vi "CycleX.vi"(0 "Devices queue":refnum<queue>, 1 "Program only changes":bool, 5 "Program during MOT loading":bool, 7 "Igor Inform String":string[](array[string]), 9 "Additional wait time (s)":dbl, 11 "error in":errorcluster) -> (8 "error out":errorcluster)   [LabVIEW 2013]
uses:
  Device/Device.lvclass
  Master Device/Master Device.lvclass
  Globals/Total Time.vi
panel:
  # "Status and timing"
  # "Igor options"
  # "Hardware control"
  # "This option starts the pulse blaster and then programs the external devices.  If the MOT loading time is not long enough for this process to complete there will be problems."
  # "When set, this option only\nasks a device to program\nitself if it's hardware image\nhas actually changed."
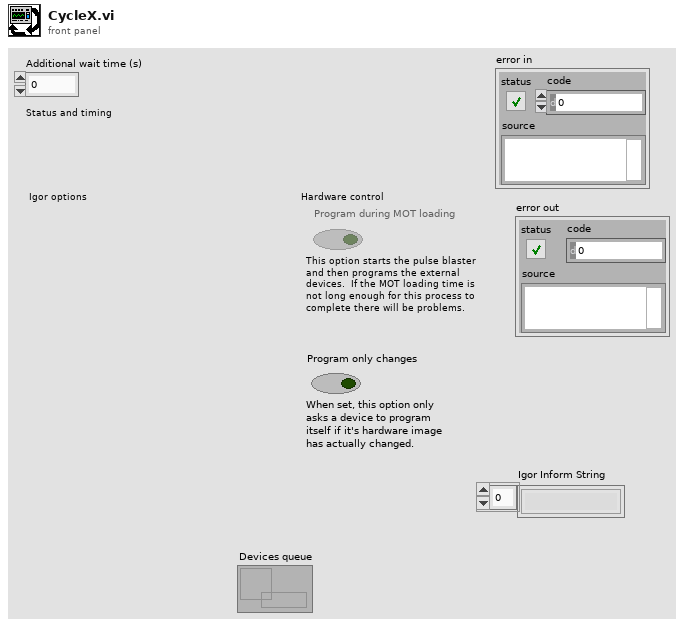
[diagram p1: front panel]
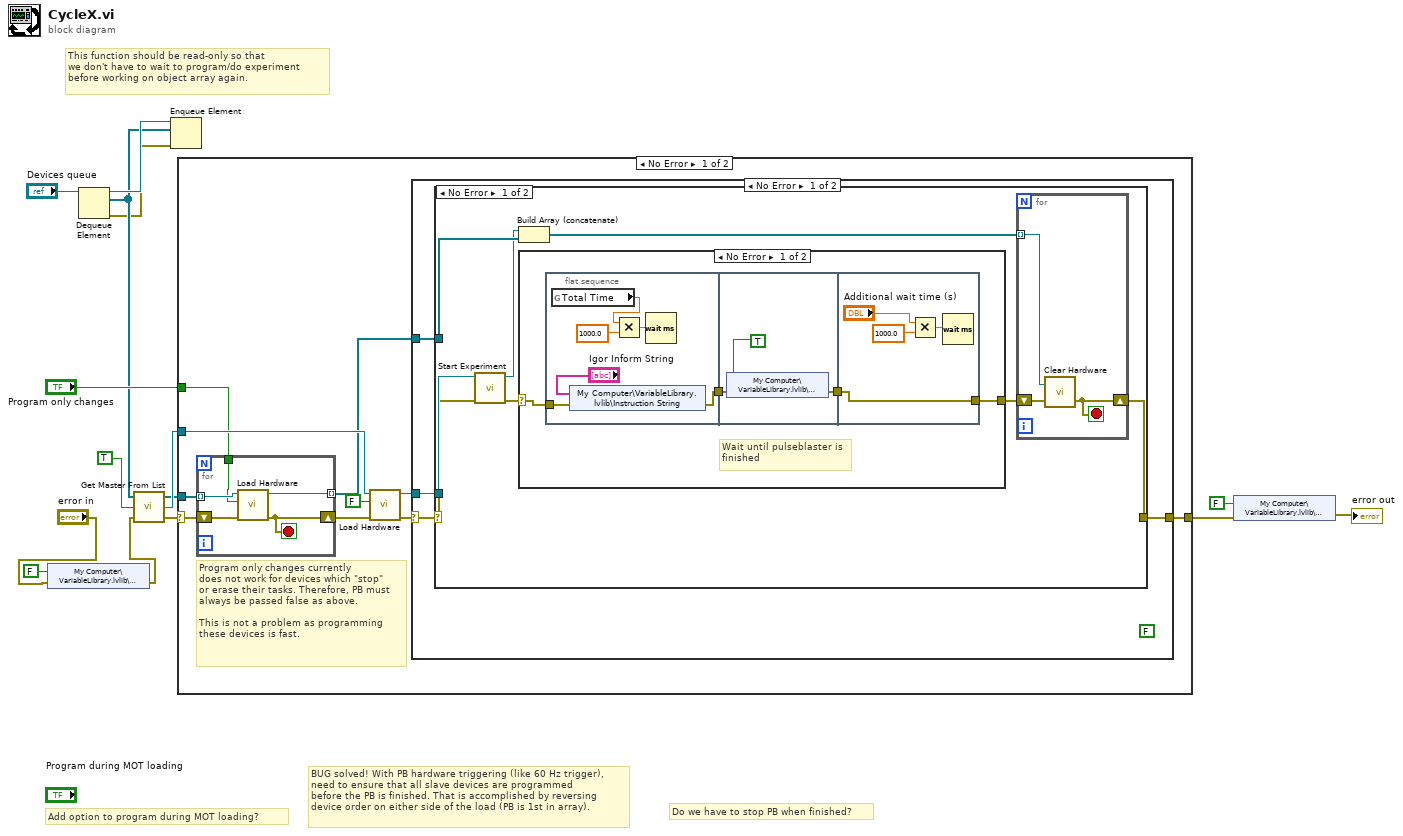
[diagram p0: block diagram]
diagram:
  # "This function should be read-only so that \nwe don't have to wait to program/do experiment \nbefore working on object array again."
  # "BUG solved! With PB hardware triggering (like 60 Hz trigger),\nneed to ensure that all slave devices are programmed\nbefore the PB is finished. That is accomplished by reversing\ndevice order on either side of the load (PB is 1st in array)."
  # "Do we have to stop PB when finished?"
  # "Add option to program during MOT loading?"
  n1 = shared-variable "My Computer\\VariableLibrary.lvlib\\CycleDone"(FALSE ("CycleDone"), error in="error in") -> (error out=w7:errorcluster)
  n2 = Dequeue Element(queue="Devices queue") -> (queue out=w10:refnum<queue>, element=w9:refnum<class "Device.lvclass">[], error out=w8:errorcluster)  [unwired: 2 in, 1 out]
  n3 = call "Get Master From List.vi"("error in"=w7, "Del From List?"=TRUE, "Device List in"=w9) -> ("error out"=w12:errorcluster, "Master Device"=w14:refnum<class "Master Device.lvclass">, "Device List out"=w13:refnum<class "Device.lvclass">[])
  n4 = Enqueue Element(queue=w10, element=w9, error in (no error)=w8) -> ()  [unwired: 1 in, 3 out]
  n5 = case shown="No Error" w12 {
    selector: w12 -> [w20 w66]
    tunnel: w14 -> [w24 _]
    tunnel: w13 -> [w23 _]
    tunnel: [w19 w66] -> w3
    tunnel: "Program only changes" -> [w17 _]
    frame No Error {
      # "Program only changes currently\ndoes not work for devices which \"stop\"\nor erase their tasks. Therefore, PB must\nalways be passed false as above.\n\nThis is not a problem as programming\nthese devices is fast."
      n6 = for {
        tunnel: w23 -> [w65] mode=indexing
        shift-right: [w63] -> w25
        shift-left: w20 -> [w64]
        tunnel: [w62] -> w22 mode=indexing
        tunnel: w17 -> [w61]
        stop <- w63 stop-if-true
        n7 = call-dynamic "Load Hardware.vi"("error in (no error)"=w64, "Program only changes"=w61, "Device in"=w65) -> ("error out"=w63:errorcluster, "Device out"=w62:refnum<class "Device.lvclass">)  [unwired: 7 in]
      }
      n8 = call-dynamic "Load Hardware.vi"("error in (no error)"=w25, "Program only changes"=FALSE, "Master Device in"=w24) -> ("error out"=w18:errorcluster, "Master Device out"=w21:refnum<class "Master Device.lvclass">)  [unwired: 7 in]
      n9 = case shown="No Error" w18 {
        selector: w18 -> [w26 w60]
        tunnel: w22 -> [w27 _]
        tunnel: [w29 w60] -> w19
        tunnel: w21 -> [w28 _]
        frame No Error {
          (unwired) FALSE ("Del From List?")
          n10 = case shown="No Error" w26 {
            selector: w26 -> [w36 w59]
            tunnel: w28 -> [w37 _]
            tunnel: w27 -> [w34 _]
            tunnel: [w35 w59] -> w29
            frame No Error {
              n11 = call-dynamic "Start Experiment.vi"("error in (no error)"=w36, "Master Device in"=w37) -> ("error out"=w33:errorcluster, "Master Device out"=w31:refnum<class "Master Device.lvclass">)  [unwired: 8 in]
              n12 = Build Array (concatenate)(w31, w34) -> (w32:refnum<class "Device.lvclass">[])
              n13 = case shown="No Error" w33 {
                selector: w33 -> [w41 w55]
                tunnel: [w38 w55] -> w30
                frame No Error {
                  # "Wait until pulseblaster is\nfinished"
                  n14 = flat-sequence {
                    tunnel: w41 -> [w43]
                    tunnel: [w42] -> w40
                    tunnel: w40 -> [w49]
                    tunnel: [w48] -> w39
                    tunnel: w39 -> [w51]
                    tunnel: [w51] -> w38
                    frame #0 {
                      n15 = global read "Total Time.vi" "Total Time"() -> (w45:dbl)
                      n16 = shared-variable "My Computer\\VariableLibrary.lvlib\\Instruction String"("Igor Inform String", error in=w43) -> (error out=w42:errorcluster)
                      n17 = Multiply(x=w45, y=1000.0) -> (x*y=w46:dbl)
                      n18 = Wait (ms)(milliseconds to wait=w46) -> ()  [unwired: 1 out]
                    }
                    frame #1 {
                      n19 = shared-variable "My Computer\\VariableLibrary.lvlib\\CycleDone"(TRUE ("CycleDone"), error in=w49) -> (error out=w48:errorcluster)
                    }
                    frame #2 {
                      n20 = Multiply(x="Additional wait time (s)", y=1000.0) -> (x*y=w53:dbl)
                      n21 = Wait (ms)(milliseconds to wait=w53) -> ()  [unwired: 1 out]
                    }
                  }
                }
                frame Error {
                }
              }
              n22 = for {
                shift-right: [w57] -> w35
                shift-left: w30 -> [w58]
                tunnel: w32 -> [w56] mode=indexing
                stop <- w57 stop-if-true
                n23 = call-dynamic "Clear Hardware.vi"("error in (no error)"=w58, "Device in"=w56) -> ("error out"=w57:errorcluster)  [unwired: 1 out]
              }
            }
            frame Error {
            }
          }
        }
        frame Error {
        }
      }
    }
    frame Error {
    }
  }
  n24 = shared-variable "My Computer\\VariableLibrary.lvlib\\CycleDone"(FALSE ("CycleDone"), error in=w3) -> (error out=→"error out":errorcluster)
